vi "HFRR ADV v02.vi"() -> ()   [LabVIEW 2025] (continued)
                    n2446 = Array Size(array=w3448) -> (size(s)=w3447:i32)
                    n2447 = case shown="True" w3458 {
                      tunnel: w3454 -> [_ w3478]
                      tunnel: w3447 -> [_ w3471]
                      frame False {
                      }
                      frame True {
                        n2448 = Number To Decimal String(number=w3471) -> (decimal integer string=w3474:string)  [unwired: 1 in]
                        n2449 = Search/Split String(string=w3478, search string/char (-)="_(" ("regular expression")) -> (substring before match=w3476:string)  [unwired: 1 in, 2 out]
                        n2450 = Concatenate Strings(w3476, "_(" ("regular expression"), w3474, ")" ("regular expression")) -> (w3472:string)
                        n2451 = local write "FILE"(w3472) -> ()
                      }
                    }
                  }
                  frame #1 {
                    w3479 = 0.0
                    w3494 = cluster{"y":dbl, dbl, "y":dbl}[] [] ("History Data")
                    w3495 = FALSE ("Heater Button")
                    (unwired) ")!" ("string")
                    (unwired) ")" ("string")
                    w3480 = dbl[] [] ("History Data")
                    w3499 = "\r"
                    # "C:\\WinDucom\\Data\\"
                    # "C:\\LAB-IQ-NXT\\data"
                    n2452 = local write "Humidity ( %RH )"(w3479) -> ()
                    n2453 = local write "Frequency ( Hz )"(w3479) -> ()
                    n2454 = local write "Stroke 3"(w3479) -> ()
                    n2455 = local write "speedop"(0.0 ("PIDclk 2")) -> ()
                    n2456 = local write "Set Temp 2"(65.0 ("Set Temp 2")) -> ()
                    n2457 = local write "%RH"(w3479) -> ()
                    n2458 = local write "TEMP 4"(w3479) -> ()
                    n2459 = local write "AIR TEMP"(w3479) -> ()
                    n2460 = local write "clk"(0.0 ("clk")) -> ()
                    n2461 = local write "Stroke 4"(w3479) -> ()
                    n2462 = local write "COF 2"(w3479) -> ()
                    n2463 = local write "Humidity ( %RH )"(w3479) -> ()
                    n2464 = local write "TEMP"(w3479) -> ()
                    n2465 = local write "ecr 3"(w3479) -> ()
                    n2466 = local write "FF 3"(w3479) -> ()
                    n2467 = local write "FF 2"(w3479) -> ()
                    n2468 = local write "Air Temperature"(w3479) -> ()
                    n2469 = property on="Humidity ( %RH )" class="WFChart (strict)"("History Data"=w3480) -> ()  [unwired: 2 in, 2 out]
                    n2470 = property on="Coefficient of Friction" class="WFChart (strict)"("History Data"=w3480) -> ()  [unwired: 2 in, 2 out]
                    n2471 = property on="Coefficient of Friction" class="WFChart (strict)"("History Data"=w3480) -> ()  [unwired: 2 in, 2 out]
                    n2472 = property on="Frictional Force ( N )" class="WFChart (strict)"("History Data"=w3480) -> ()  [unwired: 2 in, 2 out]
                    n2473 = property on="Electrical Contact Resistance ( % ) 2" class="WFChart (strict)"("History Data"=w3480) -> ()  [unwired: 2 in, 2 out]
                    n2474 = property on="Electrical Contact Resistance ( % ) 2" class="WFChart (strict)"("History Data"=w3480) -> ()  [unwired: 2 in, 2 out]
                    n2475 = property on="Temperature ( Deg C )" class="WFChart (strict)"("History Data"=w3480) -> ()  [unwired: 2 in, 2 out]
                    n2476 = property on="Frictional Force ( N )" class="WFChart (strict)"("History Data"=w3480) -> ()  [unwired: 2 in, 2 out]
                    n2477 = property on="Coefficient of Friction" class="WFChart (strict)"("History Data"=w3480) -> ()  [unwired: 2 in, 2 out]
                    n2478 = property on="Frictional Force ( N )" class="WFChart (strict)"("History Data"=w3480) -> ()  [unwired: 2 in, 2 out]
                    n2479 = property on="Electrical Contact Resistance ( % )" class="WFChart (strict)"("History Data"=w3480) -> ()  [unwired: 2 in, 2 out]
                    n2480 = property on="Temperature ( Deg C )" class="WFChart (strict)"("History Data"=w3480) -> ()  [unwired: 2 in, 2 out]
                    n2481 = property on="Humidity ( %RH )" class="WFChart (strict)"("History Data"=w3480) -> ()  [unwired: 2 in, 2 out]
                    n2482 = property on="Air Temperature ( Deg C )" class="WFChart (strict)"("History Data"=w3480) -> ()  [unwired: 2 in, 2 out]
                    n2483 = property on="Air Temperature ( Deg C )" class="WFChart (strict)"("History Data"=w3480) -> ()  [unwired: 2 in, 2 out]
                    n2484 = property on="Stroke ( mm )" class="WFChart (strict)"("History Data"=w3494) -> ()  [unwired: 2 in, 2 out]
                    n2485 = property on="Stroke ( mm )" class="WFChart (strict)"("History Data"=w3494) -> ()  [unwired: 2 in, 2 out]
                    n2486 = local write "Humidity"(w3495) -> ()
                    n2487 = local write "Heater Button"(w3495) -> ()
                    n2488 = local read "FILE"() -> (w3490:string)
                    n2489 = disable-structure shown="Enabled" {
                      disable-tunnel: [w3533 _] -> w3482
                      frame Enabled {
                        n2490 = local read "NORMAL LOAD"() -> (w3533:dbl)
                      }
                      frame Disabled {
                      }
                    }
                    n2491 = call "file check.vi"("file name in"=w3490) -> ("error out"=w3493:errorcluster, "file name out"=w3487:string)  [unwired: 9 in]
                    n2492 = call "FILE PATH CREATION.vi"("error in"=w3493, "FILE NAME :"=w3487) -> ("FILE OUT"=w3486:path)  [unwired: 8 in, 1 out]
                    n2493 = Concatenate Strings(w3487, ".dgf" ("Substring")) -> (w3492:string)
                    n2494 = Concatenate Strings(w3487, ".duf" ("Substring")) -> (w3488:string)
                    n2495 = Multiply(x=w3482, y=1.0) -> (x*y=w3512:dbl)
                    n2496 = Build Path(base path=w3486, name or relative path=w3492) -> (appended path=w3485:path)
                    n2497 = Build Path(base path=w3486, name or relative path=w3488) -> (appended path=w3484:path)
                    n2498 = Number To Fractional String(number=w3512, width (-)=i16 5, precision (6)=i16 2) -> (F-format string=w3520:string)  [unwired: 1 in]
                    n2499 = local read "tested by"() -> (w3481:string)
                    n2500 = local read "Fuel Discription :"() -> (w3508:string)
                    n2501 = local read "Batch Ref Num :"() -> (w3497:string)
                    n2502 = Get Date/Time String(date format (0)=enum16{"short", "long", "abbreviated"}."short") -> (date string=w3531:string, time string=w3528:string)  [unwired: 2 in]
                    n2503 = local read "Remarks :"() -> (w3507:string)
                    n2504 = Concatenate Strings("Load :- " ("Substring"), w3520, " grams ," ("Substring")) -> (w3519:string)
                    n2505 = local read "String 41"() -> (w3500:string)
                    n2506 = Concatenate Strings(w3508) -> (w3509:string)
                    n2507 = Concatenate Strings(w3497) -> (w3496:string)
                    n2508 = Concatenate Strings(w3481) -> (w3503:string)
                    n2509 = Concatenate Strings("(" ("Substring"), w3531, ")" ("Substring"), w3528) -> (w3502:string)
                    "concatenated string" <- w3502
                    n2510 = Concatenate Strings(w3507, "," ("string")) -> (w3506:string)
                    n2511 = Concatenate Strings("  TIME;      COF;       STROKE;     AIR TEMP;  TEMP;  HUMIDITY;  ECR; PID-OUT; FREQUENCY" ("Substring"), "\r") -> (w3515:string)
                    n2512 = Concatenate Strings(w3500, w3499, "Fuel Discription :-" ("Substring"), w3509, w3499, w3519, w3499, "Batch Ref Num :-" ("Substring"), w3496, w3499, " Remarks :- " ("Substring"), w3506, w3499, " Date :- " ("Substring"), w3502, w3499, "Tested By :-" ("Substring"), w3503) -> (w3513:string)
                    "REMARKS" <- w3513
                    n2513 = call <vilib>:"Write Characters To File.vi"("append to file? (new file:F)"=FALSE, "character string"=w3515, "file path (dialog if empty)"=w3485) -> ()  [unwired: 2 in, 1 out]
                    n2514 = call <vilib>:"Write Characters To File.vi"("append to file? (new file:F)"=FALSE, "character string"=w3513, "file path (dialog if empty)"=w3484) -> ()  [unwired: 2 in, 1 out]
                  }
                  frame #2 {
                    n2515 = local write "Cycles elapsed"(0 ("Cycles elapsed")) -> ()
                    n2516 = local write "cyclecount"(0 ("cyclecount")) -> ()
                    n2517 = local write "Save & Continue"(FALSE ("OK")) -> ()
                    n2518 = local write "autostrtflg"(TRUE ("autostrtflg")) -> ()
                    n2519 = local write "Save"(FALSE ("Save")) -> ()
                    n2520 = Get Date/Time In Seconds() -> (seconds since 1Jan1904=w3538:timestamp)
                    n2521 = To Double Precision Float(number=w3538) -> (double precision float=w3537:dbl)
                    n2522 = local write "acq timer"(w3537) -> ()
                    n2523 = One Button Dialog(message="Please ensure sample is mounted properly and machine is ready in all aspects for testing !", button name ("OK")="Ok") -> ()  [unwired: 1 out]
                  }
                  frame #3 {
                    n2524 = stacked-sequence {
                      frame #0 {
                        n2525 = local write "Main Dashboard Buttons"(T1."Dashboard" ("Main Dashboard Buttons")) -> ()
                        n2526 = local write "Main Tab"(T4."Acquire" ("Main Tab")) -> ()
                      }
                      frame #1 {
                        n2527 = local write "EVENT LOG"("" ("EVENT LOG")) -> ()
                      }
                      frame #2 {
                        n2528 = Wait (ms)(milliseconds to wait=u32 50) -> ()  [unwired: 1 out]
                      }
                      frame #3 {
                        n2529 = disable-structure shown="Disabled" {
                          frame Disabled {
                            n2530 = local read "EVENT LOG"() -> (w3550:string)
                            n2531 = call "Event Log.vi"("Content"="Test Details", "EVENT LOG"=w3550) -> ("EVENT LOG"=w3549:string)  [unwired: 8 in, 1 out]
                            n2532 = local write "EVENT LOG"(w3549) -> ()
                          }
                          frame Enabled {
                          }
                        }
                      }
                      frame #4 {
                        n2533 = Wait (ms)(milliseconds to wait=u32 50) -> ()  [unwired: 1 out]
                      }
                      frame #5 {
                        n2534 = local read "FILE"() -> (w3552:string)
                        n2535 = Concatenate Strings("File Name :" ("Content"), w3552) -> (w3553:string)
                        n2536 = local read "EVENT LOG"() -> (w3556:string)
                        n2537 = call "Event Log.vi"("Content"=w3553, "EVENT LOG"=w3556) -> ("EVENT LOG"=w3555:string)  [unwired: 8 in, 1 out]
                        n2538 = local write "EVENT LOG"(w3555) -> ()
                      }
                      frame #6 {
                        n2539 = Wait (ms)(milliseconds to wait=u32 50) -> ()  [unwired: 1 out]
                      }
                      frame #7 {
                        n2540 = local read "Batch Ref Num :"() -> (w3558:string)
                        n2541 = Concatenate Strings("Batch Ref No :" ("Content"), w3558) -> (w3559:string)
                        n2542 = local read "EVENT LOG"() -> (w3562:string)
                        n2543 = call "Event Log.vi"("Content"=w3559, "EVENT LOG"=w3562) -> ("EVENT LOG"=w3561:string)  [unwired: 8 in, 1 out]
                        n2544 = local write "EVENT LOG"(w3561) -> ()
                      }
                      frame #8 {
                        n2545 = Wait (ms)(milliseconds to wait=u32 50) -> ()  [unwired: 1 out]
                      }
                      frame #9 {
                        n2546 = local read "tested by"() -> (w3564:string)
                        n2547 = Concatenate Strings("Tested By :" ("Content"), w3564) -> (w3565:string)
                        n2548 = local read "EVENT LOG"() -> (w3568:string)
                        n2549 = call "Event Log.vi"("Content"=w3565, "EVENT LOG"=w3568) -> ("EVENT LOG"=w3567:string)  [unwired: 8 in, 1 out]
                        n2550 = local write "EVENT LOG"(w3567) -> ()
                      }
                      frame #10 {
                        n2551 = Wait (ms)(milliseconds to wait=u32 50) -> ()  [unwired: 1 out]
                      }
                      frame #11 {
                        n2552 = local read "TEST STANDARD"() -> (w3571:T5)
                        n2553 = case shown="\"ASTM D7688\"" w3571 {
                          tunnel: ["ASTM D6079" "ISO 12156" "ASTM D7688" "Custom"] -> w3570
                          frame "ASTM D6079", Default {
                          }
                          frame "ISO 12156" {
                          }
                          frame "ASTM D7688" {
                          }
                          frame "Custom" {
                          }
                        }
                        n2554 = Concatenate Strings("Test Standard :" ("Content"), w3570) -> (w3572:string)
                        n2555 = local read "EVENT LOG"() -> (w3575:string)
                        n2556 = call "Event Log.vi"("Content"=w3572, "EVENT LOG"=w3575) -> ("EVENT LOG"=w3574:string)  [unwired: 8 in, 1 out]
                        n2557 = local write "EVENT LOG"(w3574) -> ()
                      }
                      frame #12 {
                        n2558 = Wait (ms)(milliseconds to wait=u32 50) -> ()  [unwired: 1 out]
                      }
                      frame #13 {
                        n2559 = local read "Fuel Discription :"() -> (w3581:string)
                        n2560 = Concatenate Strings("Fuel Description :" ("Content"), w3581) -> (w3582:string)
                        n2561 = local read "EVENT LOG"() -> (w3585:string)
                        n2562 = call "Event Log.vi"("Content"=w3582, "EVENT LOG"=w3585) -> ("EVENT LOG"=w3584:string)  [unwired: 8 in, 1 out]
                        n2563 = local write "EVENT LOG"(w3584) -> ()
                      }
                      frame #14 {
                        n2564 = Wait (ms)(milliseconds to wait=u32 50) -> ()  [unwired: 1 out]
                      }
                      frame #15 {
                        n2565 = local read "Remarks :"() -> (w3587:string)
                        n2566 = Concatenate Strings("Remarks :" ("Content"), w3587) -> (w3588:string)
                        n2567 = local read "EVENT LOG"() -> (w3591:string)
                        n2568 = call "Event Log.vi"("Content"=w3588, "EVENT LOG"=w3591) -> ("EVENT LOG"=w3590:string)  [unwired: 8 in, 1 out]
                        n2569 = local write "EVENT LOG"(w3590) -> ()
                      }
                      frame #16 {
                        n2570 = Wait (ms)(milliseconds to wait=u32 50) -> ()  [unwired: 1 out]
                      }
                      frame #17 {
                        n2571 = local read "USER ID"() -> (w3593:string)
                        n2572 = Concatenate Strings("Operator ID :" ("Content"), w3593) -> (w3595:string)
                        n2573 = local read "EVENT LOG"() -> (w3597:string)
                        n2574 = call "Event Log.vi"("Content"=w3595, "EVENT LOG"=w3597) -> ("EVENT LOG"=w3596:string)  [unwired: 8 in, 1 out]
                        n2575 = local write "EVENT LOG"(w3596) -> ()
                      }
                      frame #18 {
                        n2576 = Wait (ms)(milliseconds to wait=u32 50) -> ()  [unwired: 1 out]
                      }
                      frame #19 {
                        n2577 = disable-structure shown="Disabled" {
                          frame Disabled {
                            n2578 = local read "EVENT LOG"() -> (w3601:string)
                            n2579 = call "Event Log.vi"("Content"="Test Parameter", "EVENT LOG"=w3601) -> ("EVENT LOG"=w3600:string)  [unwired: 8 in, 1 out]
                            n2580 = local write "EVENT LOG"(w3600) -> ()
                          }
                          frame Enabled {
                          }
                        }
                      }
                      frame #20 {
                        n2581 = Wait (ms)(milliseconds to wait=u32 50) -> ()  [unwired: 1 out]
                      }
                      frame #21 {
                        n2582 = local read "Set Hz"() -> (w3605:dbl)
                        n2583 = Number To Fractional String(number=w3605, precision (6)=i16 2) -> (F-format string=w3604:string)  [unwired: 2 in]
                        n2584 = Concatenate Strings("Set Frequency [Hz] :" ("Content"), w3604) -> (w3607:string)
                        n2585 = local read "EVENT LOG"() -> (w3609:string)
                        n2586 = call "Event Log.vi"("Content"=w3607, "EVENT LOG"=w3609) -> ("EVENT LOG"=w3608:string)  [unwired: 8 in, 1 out]
                        n2587 = local write "EVENT LOG"(w3608) -> ()
                      }
                      frame #22 {
                        n2588 = Wait (ms)(milliseconds to wait=u32 50) -> ()  [unwired: 1 out]
                      }
                      frame #23 {
                        n2589 = local read "NORMAL LOAD"() -> (w3612:dbl)
                        n2590 = Number To Fractional String(number=w3612, precision (6)=i16 2) -> (F-format string=w3613:string)  [unwired: 2 in]
                        n2591 = Concatenate Strings("Applied Load [grams] :" ("Content"), w3613) -> (w3615:string)
                        n2592 = local read "EVENT LOG"() -> (w3617:string)
                        n2593 = call "Event Log.vi"("Content"=w3615, "EVENT LOG"=w3617) -> ("EVENT LOG"=w3616:string)  [unwired: 8 in, 1 out]
                        n2594 = local write "EVENT LOG"(w3616) -> ()
                      }
                      frame #24 {
                        n2595 = Wait (ms)(milliseconds to wait=u32 50) -> ()  [unwired: 1 out]
                      }
                      frame #25 {
                        n2596 = local read "Set Strk"() -> (w3620:dbl)
                        n2597 = Number To Fractional String(number=w3620, precision (6)=i16 2) -> (F-format string=w3621:string)  [unwired: 2 in]
                        n2598 = Concatenate Strings("Set Stroke [mm] :" ("Content"), w3621) -> (w3623:string)
                        n2599 = local read "EVENT LOG"() -> (w3625:string)
                        n2600 = call "Event Log.vi"("Content"=w3623, "EVENT LOG"=w3625) -> ("EVENT LOG"=w3624:string)  [unwired: 8 in, 1 out]
                        n2601 = local write "EVENT LOG"(w3624) -> ()
                      }
                      frame #26 {
                        n2602 = Wait (ms)(milliseconds to wait=u32 50) -> ()  [unwired: 1 out]
                      }
                      frame #27 {
                        n2603 = local read "Set Temp"() -> (w3628:dbl)
                        n2604 = Number To Fractional String(number=w3628, precision (6)=i16 2) -> (F-format string=w3629:string)  [unwired: 2 in]
                        n2605 = Concatenate Strings("Set Temperature [deg C] :" ("Content"), w3629) -> (w3631:string)
                        n2606 = local read "EVENT LOG"() -> (w3633:string)
                        n2607 = call "Event Log.vi"("Content"=w3631, "EVENT LOG"=w3633) -> ("EVENT LOG"=w3632:string)  [unwired: 8 in, 1 out]
                        n2608 = local write "EVENT LOG"(w3632) -> ()
                      }
                      frame #28 {
                        n2609 = Wait (ms)(milliseconds to wait=u32 50) -> ()  [unwired: 1 out]
                      }
                      frame #29 {
                        n2610 = local read "Set Rh"() -> (w3636:dbl)
                        n2611 = Number To Fractional String(number=w3636, precision (6)=i16 2) -> (F-format string=w3637:string)  [unwired: 2 in]
                        n2612 = Concatenate Strings("Set Humidity [%RH] :" ("Content"), w3637) -> (w3639:string)
                        n2613 = local read "EVENT LOG"() -> (w3641:string)
                        n2614 = call "Event Log.vi"("Content"=w3639, "EVENT LOG"=w3641) -> ("EVENT LOG"=w3640:string)  [unwired: 8 in, 1 out]
                        n2615 = local write "EVENT LOG"(w3640) -> ()
                      }
                      frame #30 {
                        n2616 = Wait (ms)(milliseconds to wait=u32 50) -> ()  [unwired: 1 out]
                      }
                      frame #31 {
                        n2617 = local read "test time"() -> (w3644:dbl)
                        n2618 = Number To Fractional String(number=w3644, precision (6)=i16 1) -> (F-format string=w3645:string)  [unwired: 2 in]
                        n2619 = Concatenate Strings("Test Duration [mins] :" ("Content"), w3645) -> (w3647:string)
                        n2620 = local read "EVENT LOG"() -> (w3649:string)
                        n2621 = call "Event Log.vi"("Content"=w3647, "EVENT LOG"=w3649) -> ("EVENT LOG"=w3648:string)  [unwired: 8 in, 1 out]
                        n2622 = local write "EVENT LOG"(w3648) -> ()
                      }
                      frame #32 {
                        w3650 = dbl[] [] ("History Data")
                        w3651 = cluster{"y":dbl, dbl, "y":dbl}[] [] ("History Data")
                        w3652 = FALSE ("Visible")
                        n2623 = property on="Stroke ( mm )" class="WFChart (strict)"("History Data"=w3651) -> ()  [unwired: 2 in, 2 out]
                        n2624 = property on="Temperature ( Deg C )" class="WFChart (strict)"("History Data"=w3650) -> ()  [unwired: 2 in, 2 out]
                        n2625 = property on="Electrical Contact Resistance ( % ) 2" class="WFChart (strict)"("History Data"=w3650) -> ()  [unwired: 2 in, 2 out]
                        n2626 = property on="Coefficient of Friction" class="WFChart (strict)"("History Data"=w3650) -> ()  [unwired: 2 in, 2 out]
                        n2627 = property on="Frictional Force ( N )" class="WFChart (strict)"("History Data"=w3650) -> ()  [unwired: 2 in, 2 out]
                        n2628 = property on="Humidity ( %RH )" class="WFChart (strict)"("History Data"=w3650) -> ()  [unwired: 2 in, 2 out]
                        n2629 = property on="Coefficient of Friction" class="WFChart (strict)"("History Data"=w3650) -> ()  [unwired: 2 in, 2 out]
                        n2630 = property on="Frictional Force ( N )" class="WFChart (strict)"("History Data"=w3650) -> ()  [unwired: 2 in, 2 out]
                        n2631 = property on="Electrical Contact Resistance ( % )" class="WFChart (strict)"("History Data"=w3650) -> ()  [unwired: 2 in, 2 out]
                        n2632 = property on="Stroke ( mm )" class="WFChart (strict)"("History Data"=w3651) -> ()  [unwired: 2 in, 2 out]
                        n2633 = property on="Temperature ( Deg C )" class="WFChart (strict)"("History Data"=w3650) -> ()  [unwired: 2 in, 2 out]
                        n2634 = property on="Air Temperature ( Deg C )" class="WFChart (strict)"("History Data"=w3650) -> ()  [unwired: 2 in, 2 out]
                        n2635 = property on="Air Temperature ( Deg C )" class="WFChart (strict)"("History Data"=w3650) -> ()  [unwired: 2 in, 2 out]
                        n2636 = property on="Humidity ( %RH )" class="WFChart (strict)"("History Data"=w3650) -> ()  [unwired: 2 in, 2 out]
                        n2637 = property on="Service Password Log" class="Str"("Visible"=w3652) -> ()  [unwired: 2 in, 2 out]
                        n2638 = property on="Password 3" class="Clust (strict)"("Visible"=w3652) -> ()  [unwired: 2 in, 2 out]
                      }
                    }
                    "TEST FILE NAM,E SAVED" <- TRUE ("TEST FILE NAM,E SAVED")
                  }
                }
              }
            }
          }
        }
        n2639 = local write "Test \nStatus"(w3058) -> ()
        n2640 = local write "Save"(w3058) -> ()
        n2641 = local read "Main Tab"() -> (w3052:T4)
        n2642 = case shown="True" w3055 {
          frame False {
            n2643 = local read "Rt 3"() -> (w3101:bool)
            n2644 = case shown="True" w3101 {
              frame False {
              }
              frame True {
                n2645 = local write "Rt 3"(FALSE ("Rt 3")) -> ()
              }
            }
            "Rt" <- TRUE ("Rt")
            "Rt 2" <- FALSE ("Rt")
          }
          frame True {
            n2646 = local read "Rt"() -> (w3107:bool)
            n2647 = local write "Rt 2"(TRUE ("Rt 2")) -> ()
            n2648 = case shown="True" w3107 {
              frame False {
              }
              frame True {
                n2649 = local write "Rt"(FALSE ("Rt")) -> ()
              }
            }
            "Rt 3" <- TRUE ("Rt 3")
          }
        }
        n2650 = case shown="\"Acquire\"" w3052 {
          tunnel: w3054 -> [_ w3136]
          frame Default {
            w3135 = 0.0 ("output")
            n2651 = local write "PID-out"(w3135) -> ()
            n2652 = local write "Frequency ( Hz )"(w3135) -> ()
            n2653 = local write "STROKE Initialize"(TRUE ("STROKE Initialize")) -> ()
          }
          frame "Acquire" {
            n2654 = stacked-sequence {
              frame #0 {
                n2655 = local read "Auto Start Test"() -> (w3138:bool)
                n2656 = case shown="True" w3138 {
                  tunnel: "RUN" -> [w3159 w3162]
                  tunnel: [w3159 w3161] -> w3139
                  frame False {
                  }
                  frame True {
                    n2657 = local read "Auto Start Temp"() -> (w3160:bool)
                    n2658 = Or(x=w3162, y=w3160) -> (x .or. y?=w3161:bool)
                  }
                }
                n2659 = local read "clk"() -> (w3158:dbl)
                n2660 = local read "Save"() -> (w3154:bool)
                n2661 = Equal?(x=w3158, y=0.0) -> (x = y?=w3155:bool)
                n2662 = And(x=w3155, y=w3154) -> (x .and. y?=w3156:bool)
                n2663 = Not(x="Engage") -> (.not. x?=w3145:bool)
                n2664 = case shown="False" w3139 {
                  tunnel: [0.0 w3186] -> w3141
                  frame False {
                    (unwired) TRUE ("Visible")
                    n2665 = local read "Auto Start Test"() -> (w3166:bool)
                    n2666 = local write "Start Time"(TRUE ("Start Time")) -> ()
                    n2667 = property on="Stroke 2" class="DigNum (strict)"("Visible"=FALSE) -> ()  [unwired: 2 in, 2 out]
                    n2668 = case shown="False" w3166 {
                      frame False {
                        n2669 = property on="Heater Button" class="Bool (strict)"("DisabledEnum"=T19."Enabled" ("Disabled")) -> ()  [unwired: 2 in, 2 out]
                        n2670 = property on="Humidity" class="Bool (strict)"("DisabledEnum"=T19."Enabled" ("Disabled")) -> ()  [unwired: 2 in, 2 out]
                      }
                      frame True {
                      }
                    }
                    n2671 = case shown="False" "TestCompFlg" {
                      frame False {
                        n2672 = local read "StartFlg"() -> (w3174:bool)
                        n2673 = case shown="True" w3174 {
                          frame False {
                          }
                          frame True {
                            n2674 = stacked-sequence {
                              frame #0 {
                                n2675 = local read "EVENT LOG"() -> (w3178:string)
                                n2676 = call "Event Log.vi"("Content"="Test was interrupted", "EVENT LOG"=w3178) -> ("EVENT LOG"=w3179:string)  [unwired: 8 in, 1 out]
                                n2677 = local write "EVENT LOG"(w3179) -> ()
                                n2678 = property on="RUN" class="Bool (strict)"("Visible"=TRUE) -> ()  [unwired: 2 in, 2 out]
                                n2679 = property on="Auto Start Test" class="Bool (strict)"("Visible"=TRUE) -> ()  [unwired: 2 in, 2 out]
                              }
                              frame #1 {
                                w3182 = FALSE ("StartFlg")
                                n2680 = property on="Heater Button" class="Bool (strict)"("Val(Sgnl)"=FALSE ("Value (Signaling)")) -> ()  [unwired: 2 in, 2 out]
                                n2681 = local write "Heater Button"(w3182) -> ()
                                n2682 = local write "StartFlg"(w3182) -> ()
                                n2683 = local write "Humidity"(w3182) -> ()
                                n2684 = local write "Humidity 2"(TRUE ("Humidity")) -> ()
                              }
                              frame #2 {
                                n2685 = local write "Due Write"("VC;0" ("Command")) -> ()
                              }
                              frame #3 {
                                n2686 = Wait (ms)(milliseconds to wait=u32 1500) -> ()  [unwired: 1 out]
                              }
                              frame #4 {
                                n2687 = local write "Due Write"("HE;0" ("Command")) -> ()
                              }
                            }
                          }
                        }
                      }
                      frame True {
                      }
                    }
                    n2688 = local write "String 14"("Test will autostart once parameters reach the set value." ("String 14")) -> ()
                  }
                  frame True {
                    (unwired) FALSE ("Visible")
                    n2689 = property on="Stroke 2" class="DigNum (strict)"("Visible"=TRUE) -> ()  [unwired: 2 in, 2 out]
                    n2690 = property on="STOP 2" class="Bool (strict)"("Disabled"=u8 2) -> ()  [unwired: 2 in, 2 out]
                    n2691 = local write "String 14"(" Running....." ("String 14")) -> ()
                    n2692 = property on="Heater Button" class="Bool (strict)"("DisabledEnum"=T19."Disabled and Grayed Out" ("Disabled")) -> ()  [unwired: 2 in, 2 out]
                    n2693 = property on="Humidity" class="Bool (strict)"("DisabledEnum"=T19."Disabled and Grayed Out" ("Disabled")) -> ()  [unwired: 2 in, 2 out]
                    n2694 = case shown="True" "Start Time" {
                      selector: "Start Time" -> [_ w3205]
                      frame False {
                      }
                      frame True {
                        n2695 = Not(x=w3205) -> (.not. x?=w3204:bool)
                        n2696 = local write "Start Time"(w3204) -> ()
                        n2697 = local read "EVENT LOG"() -> (w3206:string)
                        n2698 = call "Event Log.vi"("Content"="Test in progress", "EVENT LOG"=w3206) -> ("EVENT LOG"=w3208:string)  [unwired: 8 in, 1 out]
                        n2699 = local write "EVENT LOG"(w3208) -> ()
                      }
                    }
                    n2700 = disable-structure shown="Enabled" {
                      disable-tunnel: [w3197 w3203] -> w3186
                      frame Disabled {
                        n2701 = local read "Set Hz"() -> (w3200:dbl)
                        n2702 = call <vilib>:"Uniform White Noise Waveform.vi"() -> ("signal out"=w3199:waveform(dbl))  [unwired: 10 in, 1 out]
                        n2703 = Random Number (0-1)() -> (number: 0 to 1=w3196:dbl)
                        n2704 = Add(x=w3200, y=w3199) -> (x+y=w3198:waveform(dbl))
                        n2705 = Multiply(x=ext 0.01 ("y"), y=w3196) -> (x*y=w3194:ext)
                        n2706 = Multiply(x=w3198, y=w3194) -> (x*y=w3197:waveform(ext))
                      }
                      frame Enabled {
                        n2707 = call-poly <vilib>:"Random Number (Range).vi"("lower bound (0)"=49.89, "upper bound (100)"=50.8) -> ("number"=w3203:dbl)  [unwired: 9 in]
                      }
                    }
                    "StartFlg" <- TRUE ("StartFlg")
                  }
                }
                n2708 = case shown="True" w3156 {
                  frame False {
                  }
                  frame True {
                    n2709 = local write "clk"(10.0 ("clk")) -> ()
                    n2710 = Get Date/Time In Seconds() -> (seconds since 1Jan1904=w3211:timestamp)
                    n2711 = To Double Precision Float(number=w3211) -> (double precision float=w3209:dbl)
                    n2712 = local write "acq timer"(w3209) -> ()
                    n2713 = local write "act save time"(w3209) -> ()
                  }
                }
                n2714 = call "Elapsed Time"("Time Target (s)"="Countdown", "Reset"=w3145) -> ("Elapsed Time (s)"=w3150:dbl, "Time has Elapsed"=w3148:bool)  [unwired: 10 in, 6 out]
                "Countdown 2" <- w3150
                n2715 = Subtract(x=w3150, y=2.0) -> (x-y=w3153:dbl)
                n2716 = Less?(x=w3153, y="Countdown") -> (x < y?=w3151:bool)
                n2717 = And(x=w3151, y=w3148) -> (x .and. y?=w3147:bool)
                n2718 = case shown="True" w3147 {
                  frame False {
                  }
                  frame True {
                    (unwired) dbl[] [] ("History Data")
                    n2719 = local write "Engage"(FALSE ("Engage")) -> ()
                    n2720 = local write "RUN"(TRUE ("RUN")) -> ()
                    n2721 = local read "Humidity ( %RH )"() -> (→"Rh Before":dbl)
                  }
                }
                n2722 = local read "Test \nStatus"() -> (w3143:bool)
                n2723 = Select(t=w3141, s=w3143, f=0.0) -> (s? t:f=w3142:dbl)
                n2724 = local write "Frequency ( Hz )"(w3142) -> ()
              }
              frame #1 {
                w3234 = 1000000.0 ("x")
                # "HC;1/0\nST;VALUE"
                # "Elapsed time\ncof\nstroke\nAir temp\nTemp\nHumidity"
                # "acq timer\n\nact save time"
                # "convert to microseconds"
                n2725 = local read "COUNT"() -> (w3217:i32)
                n2726 = local read "Rate"() -> (w3230:dbl)
                n2727 = Divide(x=w3234, y=w3230) -> (x/y=w3235:dbl)
                n2728 = Greater Or Equal?(x=w3217, y=250) -> (x >= y?=w3216:bool)
                n2729 = Get Date/Time In Seconds() -> (seconds since 1Jan1904=w3237:timestamp)
                n2730 = case shown="True" w3216 {
                  frame False {
                    n2731 = local read "COUNT"() -> (w3238:i32)
                    n2732 = Increment(x=w3238) -> (x+1=w3239:i32)
                    n2733 = local write "COUNT"(w3239) -> ()
                  }
                  frame True {
                    n2734 = local write "COUNT"(0 ("COUNT")) -> ()
                  }
                }
                n2735 = local read "Samplingtime 2"() -> (w3215:dbl)
                n2736 = local read "act save time"() -> (w3232:dbl)
                n2737 = Divide(x=w3235, y=w3234) -> (x/y=w3233:dbl)
                n2738 = To Double Precision Float(number=w3237) -> (double precision float=w3226:dbl)
                n2739 = Add(x=w3232, y=w3215) -> (x+y=w3231:dbl)
                n2740 = local read "acq timer"() -> (w3236:dbl)
                n2741 = local read "COUNT"() -> (w3219:i32)
                n2742 = Greater Or Equal?(x=w3226, y=w3231) -> (x >= y?=w3214:bool)
                n2743 = Multiply(x=w3233, y=w3219) -> (x*y=w3225:dbl)
                n2744 = Subtract(x=w3226, y=w3236) -> (x-y=w3228:dbl)
                n2745 = local read "Save"() -> (w3229:bool)
                n2746 = Add(x=w3228, y=w3225) -> (x+y=w3212:dbl)
                "Elapsed time 3" <- w3212
                n2747 = And(x=w3214, y=w3229) -> (x .and. y?=w3227:bool)
                n2748 = case shown="True" w3227 {
                  tunnel: w3226 -> [_ w3352]
                  tunnel: [FALSE ("Boolean 2") TRUE ("Boolean 2")] -> _
                  frame False {
                  }
                  frame True {
                    w3309 = ";" ("Substring")
                    # "Pid out/\nFreq response value"
                    n2749 = local write "act save time"(w3352) -> ()
                    n2750 = local read "LVDT STROKE"() -> (w3298:dbl)
                    n2751 = local read "Add up Stroke"() -> (w3296:dbl)
                    n2752 = local read "FF 2"() -> (→"Frictional Force ( N )" →"Frictional Force ( N )":dbl)
                    n2753 = local read "STROKE Initialize"() -> (w3291:bool)
                    n2754 = Subtract(x=w3298, y=w3296) -> (x-y=w3297:dbl)
                    n2755 = Absolute Value(x=w3297) -> (abs(x)=w3294:dbl)
                    n2756 = flat-sequence {
                      tunnel: w3294 -> [w3357]
                      tunnel: [w3356] -> w3292
                      tunnel: w3291 -> [w3354]
                      tunnel: [w3359] -> w3293
                      tunnel: w3292 -> [w3359]
                      frame #0 {
                        n2757 = call <vilib>:"Mean PtByPt.vi"("x"=w3357, "sample length"="STROKE FILTER", "initialize"=w3354) -> ("mean"=w3356:dbl)  [unwired: 1 in, 1 out]
                      }
                      frame #1 {
                        "STROKE Initialize" <- FALSE ("STROKE Initialize")
                      }
                    }
                    n2758 = local read "FILE"() -> (w3303:string)
                    n2759 = call "file check.vi"("file name in"=w3303) -> ("error out"=w3306:errorcluster, "file name out"=w3301:string)  [unwired: 9 in]
                    n2760 = call "FILE PATH CREATION.vi"("error in"=w3306, "FILE NAME :"=w3301) -> ("FILE OUT"=w3304:path)  [unwired: 8 in, 1 out]
                    n2761 = Concatenate Strings(w3301, ".dgf" ("Substring")) -> (w3305:string)
                    n2762 = Build Path(base path=w3304, name or relative path=w3305) -> (appended path=w3300:path)
                    n2763 = local read "COF 2"() -> (w3290:dbl)
                    "Coefficient of Friction" <- w3290
                    "COF 4" <- w3290
                    "Coefficient of Friction" <- w3290
                    n2764 = local read "TEMP"() -> (w3315:dbl)
                    "Temperature ( Deg C )" <- w3315
                    n2765 = local read "Humidity ( %RH )"() -> (w3289:dbl)
                    "Humidity ( %RH )" <- w3289
                    "%RH" <- w3289
                    n2766 = local read "Frequency ( Hz )"() -> (w3320:dbl)
                    n2767 = local read "LVDT STROKE DISPLAY"() -> (w3295:dbl)
                    n2768 = Number To Fractional String(number=w3295, width (-)=i16 9 ("precision (6)"), precision (6)=i16 6) -> (F-format string=w3338:string)  [unwired: 1 in]
                    n2769 = local read "Elapsed time"() -> (w3345:dbl)
                    n2770 = local read "AIR TEMP"() -> (w3288:dbl)
                    "TEMP 4" <- w3288
                    "Air Temperature ( Deg C )" <- w3288
                    n2771 = local read "PID-out"() -> (w3323:dbl)
                    n2772 = local write "Temperature ( Deg C )"(w3315) -> ()
                    n2773 = Number To Fractional String(number=w3345, width (-)=i16 14 ("precision (6)"), precision (6)=i16 3) -> (F-format string=w3347:string)  [unwired: 1 in]
                    n2774 = Number To Fractional String(number=w3290, width (-)=i16 9 ("precision (6)"), precision (6)=i16 6) -> (F-format string=w3346:string)  [unwired: 1 in]
                    n2775 = Number To Fractional String(number=w3288, width (-)=i16 9 ("precision (6)"), precision (6)=i16 3) -> (F-format string=w3337:string)  [unwired: 1 in]
                    n2776 = Number To Fractional String(number=w3315, width (-)=i16 9 ("precision (6)"), precision (6)=i16 3) -> (F-format string=w3334:string)  [unwired: 1 in]
                    n2777 = Number To Fractional String(number=w3289, width (-)=i16 9 ("precision (6)"), precision (6)=i16 3) -> (F-format string=w3331:string)  [unwired: 1 in]
                    n2778 = Number To Fractional String(number=0.0, width (-)=i16 9 ("precision (6)"), precision (6)=i16 3) -> (F-format string=w3328:string)  [unwired: 1 in]
                    n2779 = Number To Fractional String(number=w3323, width (-)=i16 9 ("precision (6)"), precision (6)=i16 3) -> (F-format string=w3324:string)  [unwired: 1 in]
                    n2780 = Number To Fractional String(number=w3320, width (-)=i16 9 ("precision (6)"), precision (6)=i16 3) -> (F-format string=w3319:string)  [unwired: 1 in]
                    n2781 = Bundle("y"=1.02, "LVDT STROKE DISPLAY"=w3295, "y"=0.98) -> (w3314:T31)  [unwired: 1 in]
                    n2782 = Number To Fractional String(number="Ambient Humidity :", width (-)=i16 9 ("precision (6)"), precision (6)=i16 6) -> (F-format string=w3307:string)  [unwired: 1 in]
                    n2783 = local write "Humidity ( %RH )"(w3289) -> ()
                    n2784 = local write "Humidity ( %RH )"(w3289) -> ()
                    n2785 = local read "RUN"() -> (w3313:bool)
                    n2786 = case shown="True" w3313 {
                      tunnel: w3314 -> [_ w3363]
                      tunnel: w3295 -> [_ w3362]
                      tunnel: w3295 -> [_ w3360]
                      tunnel: w3295 -> [_ w3361]
                      frame False {
                      }
                      frame True {
                        "Stroke ( mm )" <- w3363
                        "Stroke ( mm )" <- w3363
                        "Stroke 4" <- w3362
                        "Stroke 3" <- w3360
                        "Stroke 2" <- w3361
                        "measured_stroke" <- w3360
                      }
                    }
                    n2787 = local write "Air Temperature ( Deg C )"(w3288) -> ()
                    n2788 = local write "Air Temperature"(w3288) -> ()
                    n2789 = Concatenate Strings(w3347, w3309, w3346, w3309, w3338, w3309, w3337, w3309, w3334, w3309, w3331, w3309, w3328, w3309, w3324, w3309, w3319, w3309, w3307, "\r") -> (w3344:string)
                    n2790 = call <vilib>:"Write Characters To File.vi"("append to file? (new file:F)"=TRUE, "character string"=w3344, "file path (dialog if empty)"=w3300) -> ()  [unwired: 2 in, 1 out]
                    "refresh flag" <- TRUE ("refresh flag")
                    "LVDT STROKE Actual" <- w3293
                  }
                }
                n2791 = Divide(x=w3212, y=60.0) -> (x/y=w3223:dbl)
                n2792 = local read "Test \nStatus"() -> (w3213:bool)
                n2793 = local read "clk"() -> (w3220:dbl)
                n2794 = Equal?(x=w3220, y=10.0) -> (x = y?=w3222:bool)
                n2795 = case shown="True" w3213 {
                  tunnel: w3223 -> [_ w3248]
                  tunnel: w3228 -> [_ w3256]
                  tunnel: w3222 -> [_ w3252]
                  tunnel: w3212 -> [_ _]
                  tunnel: w3226 -> [w3242 _]
                  frame False {
                    n2796 = local write "acq timer"(w3242) -> ()
                    n2797 = local write "Test Duration Status"(0.0 ("Test Duration Status")) -> ()
                  }
                  frame True {
                    n2798 = local read "DEMO MODE"() -> (w3243:bool)
                    n2799 = case shown="True" w3243 {
                      tunnel: [w3257 w3258] -> w3247
                      frame False {
                        n2800 = local read "test time"() -> (w3257:dbl)
                      }
                      frame True {
                        n2801 = local read "DEMO TIME IN MIN"() -> (w3258:dbl)
                      }
                    }
                    n2802 = local read "Set Hz"() -> (w3253:dbl)
                    n2803 = local write "Elapsed time"(w3248) -> ()
                    n2804 = Multiply(x=w3256, y=w3253) -> (x*y=w3255:dbl)
                    n2805 = case shown="False" w3252 {
                      tunnel: w3255 -> [w3259 _]
                      tunnel: [w3259 1.0] -> _
                      frame False {
                        n2806 = local write "Cycles elapsed"(w3259) -> ()
                      }
                      frame True {
                      }
                    }
                    n2807 = Greater?(x=w3248, y=w3247) -> (0:w3254:bool)
                    n2808 = Subtract(x=w3247, y=w3248) -> (x-y=w3246:dbl)
                    n2809 = Multiply(x=w3246, y=60.0) -> (x*y=w3245:dbl)
                    n2810 = local write "Time Remaining"(w3245) -> ()
                    n2811 = local write "Remaining Time"(w3245) -> ()
                    n2812 = case shown="True" w3254 {
                      frame False {
                      }
                      frame True {
                        n2813 = stacked-sequence {
                          frame #0 {
                            w3264 = T19."Enabled" ("Disabled")
                            w3263 = FALSE ("TEST FILE NAM,E SAVED")
                            w3265 = "" ("FILE")
                            w3266 = TRUE ("Visible")
                            n2814 = local write "Humidity"(FALSE ("Humidity")) -> ()
                            n2815 = local write "RUN"(FALSE ("OK Button 2")) -> ()
                            n2816 = local write "Heater Button"(FALSE ("Heater Button")) -> ()
                            n2817 = local write "Auto Start Test"(FALSE ("Auto Start Test")) -> ()
                            n2818 = local write "TestCompFlg"(TRUE ("StpFlg")) -> ()
                            n2819 = local read "Humidity ( %RH )"() -> (→"Rh After":dbl)
                            n2820 = property on="STOP 2" class="Bool (strict)"("Disabled"=u8 0) -> ()  [unwired: 2 in, 2 out]
                            n2821 = local read "EVENT LOG"() -> (w3271:string)
                            n2822 = call "Event Log.vi"("Content"="Test Completed", "EVENT LOG"=w3271) -> ("EVENT LOG"=w3270:string)  [unwired: 8 in, 1 out]
                            n2823 = property on="RUN" class="Bool (strict)"("Visible"=w3266) -> ()  [unwired: 2 in, 2 out]
                            n2824 = property on="Auto Start Test" class="Bool (strict)"("Visible"=w3266) -> ()  [unwired: 2 in, 2 out]
                            n2825 = local write "Batch Ref Num :"(w3265) -> ()
                            n2826 = local write "FILE"(w3265) -> ()
                            n2827 = local write "EVENT LOG"(w3270) -> ()
                            n2828 = local write "TEST FILE NAM,E SAVED"(w3263) -> ()
                            n2829 = local write "Fuel Discription :"(w3265) -> ()
                            n2830 = local write "START TEMP"(w3263) -> ()
                            n2831 = local write "Remarks :"(w3265) -> ()
                            n2832 = local write "Main Dashboard Buttons"(T1."Imaging" ("Main Dashboard Buttons")) -> ()
                            n2833 = local write "Main Tab"(T4."Adv Scar" ("Main Tab")) -> ()
                            n2834 = property on="FRICVALZ 2" class="Bool (strict)"("DisabledEnum"=w3264) -> ()  [unwired: 2 in, 2 out]
                            n2835 = property on="FRICVALZ 3" class="Bool (strict)"("DisabledEnum"=w3264) -> ()  [unwired: 2 in, 2 out]
                            n2836 = property on="FRICVALZ 4" class="Bool (strict)"("DisabledEnum"=w3264) -> ()  [unwired: 2 in, 2 out]
                          }
                          frame #1 {
                            n2837 = Wait (ms)(milliseconds to wait=u32 2000) -> ()  [unwired: 1 out]
                          }
                          frame #2 {
                            n2838 = local write "Due Write"("VC;0") -> ()
                          }
                          frame #3 {
                            n2839 = Wait (ms)(milliseconds to wait=u32 2000) -> ()  [unwired: 1 out]
                          }
                          frame #4 {
                            n2840 = local write "Due Write"("VC;0") -> ()
                          }
                          frame #5 {
                            n2841 = Wait (ms)(milliseconds to wait=u32 2000) -> ()  [unwired: 1 out]
                          }
                          frame #6 {
                            n2842 = local write "Due Write"("ST;0") -> ()
                          }
                          frame #7 {
                            n2843 = local write "measured_stroke"(0.0 ("measured_stroke")) -> ()
                            n2844 = Wait (ms)(milliseconds to wait=u32 1500) -> ()  [unwired: 1 out]
                          }
                          frame #8 {
                            n2845 = local write "Due Write"("HE;0") -> ()
                            n2846 = local write "Humidity 2"(TRUE ("Humidity")) -> ()
                          }
                        }
                      }
                    }
                    n2847 = Divide(x=w3248, y=w3247) -> (x/y=w3251:dbl)
                    n2848 = Multiply(x=w3251, y=100.0) -> (x*y=w3249:dbl)
                    n2849 = local write "Test Duration Status"(w3249) -> ()
                  }
                }
              }
              frame #2 {
                n2850 = case shown="True" "Heater Button" {
                  tunnel: [0.0 ("output") w3386] -> w3364
                  frame False {
                    w3367 = TRUE ("tmpchk")
                    n2851 = local read "TEMP"() -> (w3368:dbl)
                    n2852 = local write "Temp ini"(w3368) -> ()
                    n2853 = local write "Reset 4"(w3367) -> ()
                    n2854 = local write "tmpchk"(w3367) -> ()
                    n2855 = local write "reinit"(TRUE ("reinit")) -> ()
                    n2856 = local write "manual temp log"(TRUE ("manual temp log")) -> ()
                  }
                  frame True {
                    # "Logic to turn off\nthe heater when \ntemp is not rising.\nTime - 60 sec\nDelta t- 5°c"
                    n2857 = local read "Temp ini"() -> (w3375:dbl)
                    n2858 = local read "Auto Start Test"() -> (w3371:bool)
                    n2859 = Less?(x=w3375, y=53.0) -> (x < y?=w3373:bool)
                    n2860 = case shown="False" w3371 {
                      frame False {
                        n2861 = local read "Set Temp"() -> (w3395:dbl)
                        n2862 = local read "TEMP"() -> (w3394:dbl)
                        n2863 = Subtract(x=w3395, y=w3394) -> (x-y=w3393:dbl)
                        n2864 = Absolute Value(x=w3393) -> (abs(x)=w3392:dbl)
                        n2865 = Less?(x=w3392, y=0.5) -> (x < y?=w3390:bool)
                        n2866 = case shown="True" w3390 {
                          tunnel: "manual temp log" -> [_ w3396]
                          frame False {
                          }
                          frame True {
                            n2867 = case shown="True" w3396 {
                              selector: w3396 -> [_ w3397]
                              frame False {
                              }
                              frame True {
                                # "#Event log"
                                n2868 = Not(x=w3397) -> (.not. x?=w3398:bool)
                                n2869 = local write "manual temp log"(w3398) -> ()
                                n2870 = local read "EVENT LOG"() -> (w3401:string)
                                n2871 = call "Event Log.vi"("Content"="Target Temperature reached", "EVENT LOG"=w3401) -> ("EVENT LOG"=w3400:string)  [unwired: 8 in, 1 out]
                                n2872 = local write "EVENT LOG"(w3400) -> ()
                              }
                            }
                          }
                        }
                      }
                      frame True {
                        n2873 = local write "manual temp log"(TRUE ("manual temp log")) -> ()
                      }
                    }
                    n2874 = And(x="tmpchk", y=w3373) -> (x .and. y?=w3376:bool)
                    n2875 = case shown="True" w3376 {
                      frame False {
                      }
                      frame True {
                        n2876 = call "Elapsed Time8"("Time Target (s)"=300.0, "Reset"="Reset 4") -> ("Time has Elapsed"=w3403:bool)  [unwired: 10 in, 7 out]
                        n2877 = flat-sequence {
                          tunnel: w3403 -> [_]
                          frame #0 {
                            n2878 = local write "Reset 4"(FALSE ("Reset 4")) -> ()
                          }
                        }
                        n2879 = case shown="True" w3403 {
                          frame False {
                          }
                          frame True {
                            n2880 = local read "Temp ini"() -> (w3410:dbl)
                            n2881 = Add(x=w3410, y=5.0) -> (x+y=w3408:dbl)
                            n2882 = local read "TEMP"() -> (w3411:dbl)
                            n2883 = Greater?(x=w3411, y=w3408) -> (0:w3409:bool)
                            n2884 = case shown="False" w3409 {
                              frame False {
                                n2885 = local write "Heater Button"(FALSE ("Heater Button")) -> ()
                              }
                              frame True {
                                n2886 = local write "tmpchk"(FALSE ("tmpchk")) -> ()
                              }
                            }
                          }
                        }
                      }
                    }
                    n2887 = local read "Set Temp"() -> (w3384:dbl)
                    n2888 = local read "TEMP"() -> (w3378:dbl)
                    n2889 = call-poly <vilib>:"PID.vi"("reinitialize? (F)"="reinit", "dt (s)"=-1.0, "process variable"=w3378, "setpoint"=w3384) -> ("output"=w3381:dbl)  [unwired: 6 in, 1 out]
                    n2890 = Subtract(x=w3384, y=w3378) -> (x-y=w3385:dbl)
                    n2891 = Add(x=w3384, y=0.5) -> (x+y=w3382:dbl)
                    n2892 = Greater Or Equal?(x=w3378, y=w3382) -> ()  [unwired: 1 out]
                    n2893 = Select(t=0.0, s=FALSE, f=w3381) -> (s? t:f=w3380:dbl)
                    "PID output" <- w3380
                    n2894 = flat-sequence {
                      tunnel: w3380 -> [w3414]
                      tunnel: [w3414] -> w3386
                      frame #0 {
                        n2895 = local write "reinit"(FALSE ("reinit")) -> ()
                      }
                    }
                    n2896 = Bundle(w3385, "output"=w3380, "TEMP"=w3378) -> ()  [unwired: 1 in, 1 out]
                  }
                }
                "PID-out" <- w3364
              }
              frame #3 {
                n2897 = local read "TEMP"() -> (w3416:dbl)
                n2898 = Greater Or Equal?(x=w3416, y="Set Temp 2") -> (x >= y?=w3421:bool)
                n2899 = case shown="True" w3421 {
                  tunnel: [FALSE TRUE] -> w3419
                  frame False {
                  }
                  frame True {
                  }
                }
                "Status 13" <- w3419
                n2900 = And(x=w3419, y="trip1 8") -> (x .and. y?=w3418:bool)
                n2901 = case shown="True" w3418 {
                  frame False {
                    n2902 = local write "Heater Trip Temp"(TRUE ("Heater Trip Temp")) -> ()
                  }
                  frame True {
                    w3424 = FALSE ("OK Button 2")
                    n2903 = case shown="True" "Heater Trip Temp" {
                      selector: "Heater Trip Temp" -> [_ w3426]
                      frame False {
                      }
                      frame True {
                        n2904 = Not(x=w3426) -> (.not. x?=w3425:bool)
                        n2905 = local read "EVENT LOG"() -> (w3429:string)
                        n2906 = local write "Heater Trip Temp"(w3425) -> ()
                        n2907 = call "Event Log.vi"("Content"="Heater Trip", "EVENT LOG"=w3429) -> ("EVENT LOG"=w3428:string)  [unwired: 8 in, 1 out]
                        n2908 = local write "EVENT LOG"(w3428) -> ()
                      }
                    }
                    n2909 = local write "RUN"(w3424) -> ()
                    n2910 = property on="Auto Start Test" class="Bool (strict)"("Value"=w3424) -> ()  [unwired: 2 in, 2 out]
                    n2911 = local write "Heater Button"(w3424) -> ()
                  }
                }
              }
            }
            n2912 = case shown="False" w3136 {
              frame False {
                n2913 = disable-structure shown="Disabled" {
                  frame Disabled {
                    n2914 = stacked-sequence {
                      frame #0 {
                        n2915 = local write "RUN"(FALSE ("OK Button 2")) -> ()
                      }
                      frame #1 {
                      }
                    }
                  }
                  frame Enabled {
                  }
                }
              }
              frame True {
              }
            }
          }
        }
        n2916 = local read "Reset Graph"() -> (w3051:bool)
        n2917 = case shown="True" w3051 {
          selector: w3051 -> [_ w3061]
          frame False {
          }
          frame True {
            w3075 = 0.0 ("X Scale.Range:Maximum")
            n2918 = Not(x=w3061) -> (.not. x?=w3060:bool)
            n2919 = local write "Reset Graph"(w3060) -> ()
            n2920 = property on="Electrical Contact Resistance ( % )" class="WFChart (strict)"("XScale.Maximum"=600.0 ("X Scale.Range:Maximum"), "XScale.Minimum"=0.0 ("X Scale.Range:Minimum"), "YScale.Maximum"=100.0 ("Y Scale.Range:Maximum"), "YScale.Minimum"=0.0 ("Y Scale.Range:Minimum")) -> ()  [unwired: 2 in, 2 out]
            n2921 = property on="Frictional Force ( N )" class="WFChart (strict)"("XScale.Maximum"=600.0 ("X Scale.Range:Maximum"), "XScale.Minimum"=0.0 ("X Scale.Range:Minimum"), "YScale.Maximum"=100.0 ("Y Scale.Range:Maximum"), "YScale.Minimum"=0.0 ("Y Scale.Range:Minimum")) -> ()  [unwired: 2 in, 2 out]
            n2922 = property on="Temperature ( Deg C )" class="WFChart (strict)"("XScale.Maximum"=600.0 ("X Scale.Range:Maximum"), "XScale.Minimum"=0.0 ("X Scale.Range:Minimum"), "YScale.Maximum"=100.0 ("Y Scale.Range:Maximum"), "YScale.Minimum"=0.0 ("Y Scale.Range:Minimum")) -> ()  [unwired: 2 in, 2 out]
            n2923 = property on="Stroke ( mm )" class="WFChart (strict)"("XScale.Maximum"=600.0 ("X Scale.Range:Maximum"), "XScale.Minimum"=0.0 ("X Scale.Range:Minimum"), "YScale.Maximum"=100.0 ("Y Scale.Range:Maximum"), "YScale.Minimum"=0.0 ("Y Scale.Range:Minimum")) -> ()  [unwired: 2 in, 2 out]
            n2924 = property on="Coefficient of Friction" class="WFChart (strict)"("XScale.Maximum"=600.0 ("X Scale.Range:Maximum"), "XScale.Minimum"=0.0 ("X Scale.Range:Minimum"), "YScale.Maximum"=100.0 ("Y Scale.Range:Maximum"), "YScale.Minimum"=0.0 ("Y Scale.Range:Minimum")) -> ()  [unwired: 2 in, 2 out]
            n2925 = property on="Electrical Contact Resistance ( % ) 2" class="WFChart (strict)"("XScale.Minimum"=0.0 ("X Scale.Range:Minimum"), "XScale.Maximum"=600.0 ("X Scale.Range:Maximum"), "YScale.Minimum"=0.0 ("Y Scale.Range:Minimum"), "YScale.Maximum"=100.0 ("Y Scale.Range:Maximum")) -> ()  [unwired: 2 in, 2 out]
            n2926 = property on="Temperature ( Deg C )" class="WFChart (strict)"("XScale.Minimum"=0.0 ("X Scale.Range:Minimum"), "XScale.Maximum"=600.0 ("X Scale.Range:Maximum"), "YScale.Minimum"=0.0 ("Y Scale.Range:Minimum"), "YScale.Maximum"=100.0 ("Y Scale.Range:Maximum")) -> ()  [unwired: 2 in, 2 out]
            n2927 = property on="Coefficient of Friction" class="WFChart (strict)"("XScale.Minimum"=0.0 ("X Scale.Range:Minimum"), "XScale.Maximum"=600.0 ("X Scale.Range:Maximum"), "YScale.Maximum"=1.0 ("X Scale.Range:Minimum"), "YScale.Minimum"=0.0 ("X Scale.Range:Minimum")) -> ()  [unwired: 2 in, 2 out]
            n2928 = property on="Frictional Force ( N )" class="WFChart (strict)"("XScale.Maximum"=600.0 ("X Scale.Range:Maximum"), "XScale.Minimum"=w3075, "YScale.Maximum"=10.0 ("Y Scale.Range:Maximum"), "YScale.Minimum"=w3075) -> ()  [unwired: 2 in, 2 out]
            n2929 = property on="Stroke ( mm )" class="WFChart (strict)"("XScale.Maximum"=600.0 ("X Scale.Range:Maximum"), "XScale.Minimum"=0.0 ("X Scale.Range:Minimum"), "YScale.Maximum"=100.0 ("Y Scale.Range:Maximum"), "YScale.Minimum"=0.0 ("Y Scale.Range:Minimum")) -> ()  [unwired: 2 in, 2 out]
          }
        }
      }
      frame "Compare Files" {
        # "Elapsed time\ncof\nstroke\nAir temp\nTemp\nHumidity"
        n2930 = case shown="True" "RSTV1 2" {
          frame False {
          }
          frame True {
            n2931 = property on="Humidity ( %RH )" class="XYGraph (strict)"("Y Scale.Display Format:Precision"=u8 0 ("Y Scale.Format & Precision:Precision")) -> ()  [unwired: 2 in, 2 out]
            n2932 = property on="Humidity ( %RH )" class="XYGraph (strict)"("X Scale.Range:Minimum"=0.0, "X Scale.Range:Maximum"=75.0, "Y Scale.Range:Minimum"=48.0, "Y Scale.Range:Maximum"=58.0) -> ()  [unwired: 2 in, 2 out]
          }
        }
        n2933 = case shown="True" "RST CP 2" {
          frame False {
          }
          frame True {
            n2934 = property on="XY Graph 13" class="XYGraph (strict)"("Y Scale.Display Format:Precision"=u8 0 ("Y Scale.Format & Precision:Precision")) -> ()  [unwired: 2 in, 2 out]
            n2935 = property on="XY Graph 13" class="XYGraph (strict)"("X Scale.Range:Minimum"=0.0, "X Scale.Range:Maximum"=75.0, "Y Scale.Range:Minimum"=0.0, "Y Scale.Range:Maximum"=100.0) -> ()  [unwired: 2 in, 2 out]
          }
        }
        n2936 = case shown="True" "RST CP" {
          frame False {
          }
          frame True {
            n2937 = property on="Sample Temperature ( °C )" class="XYGraph (strict)"("Y Scale.Display Format:Precision"=u8 2 ("Y Scale.Format & Precision:Precision")) -> ()  [unwired: 2 in, 2 out]
